vi "Load Plugin Action.vi"(7 "plugin path":path, 8 "error in (no error)":errorcluster, 9 "Unique Name":string, 10 "Plugin":T1, 11 "Launcher in":refnum<class "CIFPluginManager.lvclass">) -> (0 "error out":errorcluster, 3 "Launcher out":refnum<class "CIFPluginManager.lvclass">)   [LabVIEW 2021, in "CIFPluginManager.lvclass"]
doc: "This performs the loading action using VI Server. Because this process can be slow it is moved outside of the Load Plugin Prepare process. The prepare will detect most common configuration errors. This allows the UI to get any configuration errors returned but not need to wait for the full load to complete."
uses:
  CIFPluginManager.lvclass
  typedef/Discovered Plugin.ctl
  CIFCore/Common/Typedef/Version.ctl
  typedef/Plugin Metadata.ctl
  typedef/Plugin Management Data.ctl
  <vilib>/gRPC/LabVIEW gRPC Library/Shared/grpcId.ctl
  gRPC/CIF_Manager_server/RPC Messages/cif_plugincore_StatusData.ctl
  gRPC/CIF_Manager_server/RPC Messages/cif_plugincore_StatusData_State.ctl
  gRPC/CIF_Manager_server/RPC Messages/cif_plugincore_TimingStatistics.ctl
  gRPC/CIF_Manager_server/RPC Messages/cif_common_TimingStats.ctl
  gRPC/CIF_Manager_server/RPC Messages/cif_plugincore_FifoStatistics.ctl
  gRPC/CIF_Manager_server/RPC Messages/cif_plugincore_Error.ctl
  gRPC/CIF_Manager_server/RPC Messages/cif_plugincore_MonitorDoubles.ctl
  gRPC/CIF_Manager_server/RPC Messages/cif_plugincore_MonitorU64.ctl
  gRPC/CIF_Manager_server/RPC Messages/cif_plugincore_MonitorI64.ctl
  CIFPluginManager.lvclass/CIFPluginManager.ctl
  <vilib>/CIF Foundation/CIF Utilities/Time/System Time/LabVIEW Time to TAI Time.vi
  CIFCore/Common/CIFCoreCommon.lvlib
  <vilib>/gRPC/LabVIEW gRPC Library/grpc-lvsupport-release.lvlib
  gRPC/CIF_Manager_server/CIF_Manager_server.lvlib
  <vilib>/CIF Foundation/CIF Utilities/Time/Time_CIF_U.lvlib
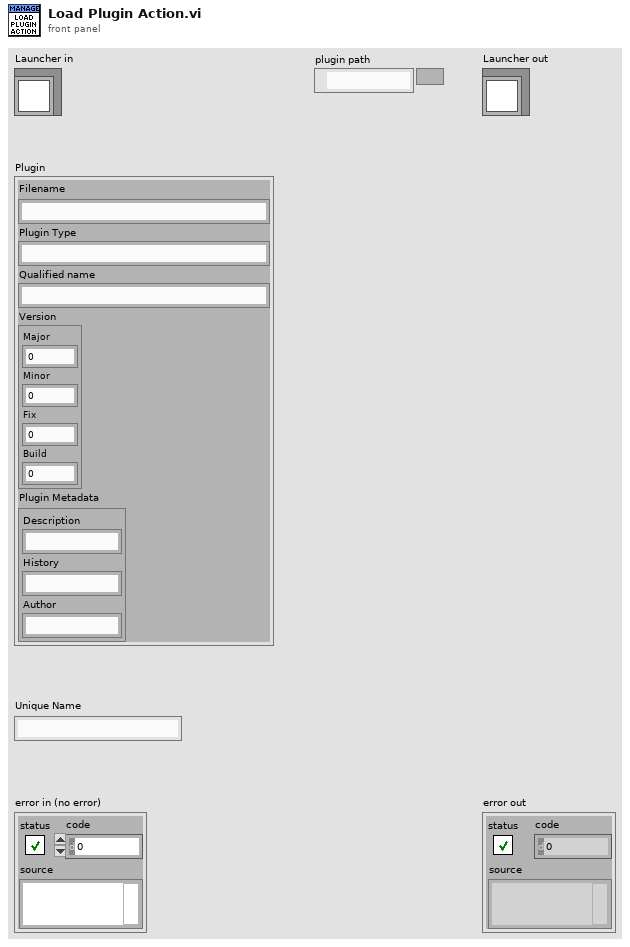
[diagram p1: front panel]
types:
  T1 = typedef "CIFPluginManager.lvclass/Discovered Plugin.ctl" = cluster{"Filename":string, "Plugin Type":string, "Qualified name":string, "Version":T2, "Plugin Metadata":T3}
  T2 = typedef "CIFCoreCommon.lvlib/Version.ctl" = cluster{"Major":i32, "Minor":i32, "Fix":i32, "Build":i32}
  T3 = typedef "CIFPluginManager.lvclass/Plugin Metadata.ctl" = cluster{"Description":string, "History":string, "Author":string}
  T4 = typedef "CIFPluginManager.lvclass/Plugin Management Data.ctl" = cluster{"vi reference":refnum<vi>, "gRPC ID":T5, "Plugin Type":string, "Unique Name":string, "gRPC Port":i32, "Version":T2, "Load Timestamp":i64, "Unload Timestamp":i64, "Unloading":bool, "Ready for removal":bool, "status":T6}
  T5 = typedef "grpc-lvsupport-release.lvlib/grpcId.ctl" = u64
  T6 = typedef "CIF_Manager_server.lvlib/cif_plugincore_StatusData.ctl" = cluster{"state":T7, "timing_statistics":T8, "fifo_statistics":T10, "error":T11, "monitor_doubles":T12, "monitor_u64s":T13, "monitor_i64s":T14}
  T7 = typedef "CIF_Manager_server.lvlib/cif_plugincore_StatusData_State.ctl" = enum32{"NULL", "CREATING", "LISTENING", "RUNNING", "CLEANINGUP", "DESTROYING"}
  T8 = typedef "CIF_Manager_server.lvlib/cif_plugincore_TimingStatistics.ctl" = cluster{"period":T9, "wake_error":T9, "execute":T9, "housekeep":T9, "idle":T9, "cleanup":T9, "custom_1":T9, "custom_2":T9}
  T9 = typedef "CIF_Manager_server.lvlib/cif_common_TimingStats.ctl" = cluster{"max":i64, "min":i64, "avg":dbl}
  T10 = typedef "CIF_Manager_server.lvlib/cif_plugincore_FifoStatistics.ctl" = cluster{"from_t0":T9, "from_previous_plugin":T9, "output_error":T9}
  T11 = typedef "CIF_Manager_server.lvlib/cif_plugincore_Error.ctl" = cluster{"status":bool, "code":i32}
  T12 = typedef "CIF_Manager_server.lvlib/cif_plugincore_MonitorDoubles.ctl" = cluster{"double_1":dbl, "double_2":dbl, "double_3":dbl, "double_4":dbl}
  T13 = typedef "CIF_Manager_server.lvlib/cif_plugincore_MonitorU64.ctl" = cluster{"u64_1":u64, "u64_2":u64, "u64_3":u64, "u64_4":u64}
  T14 = typedef "CIF_Manager_server.lvlib/cif_plugincore_MonitorI64.ctl" = cluster{"i64_1":i64, "i64_2":i64, "i64_3":i64, "i64_4":i64}
  T15 = typedef "Plugin Management Data Map.ctl" = map{string, T4}
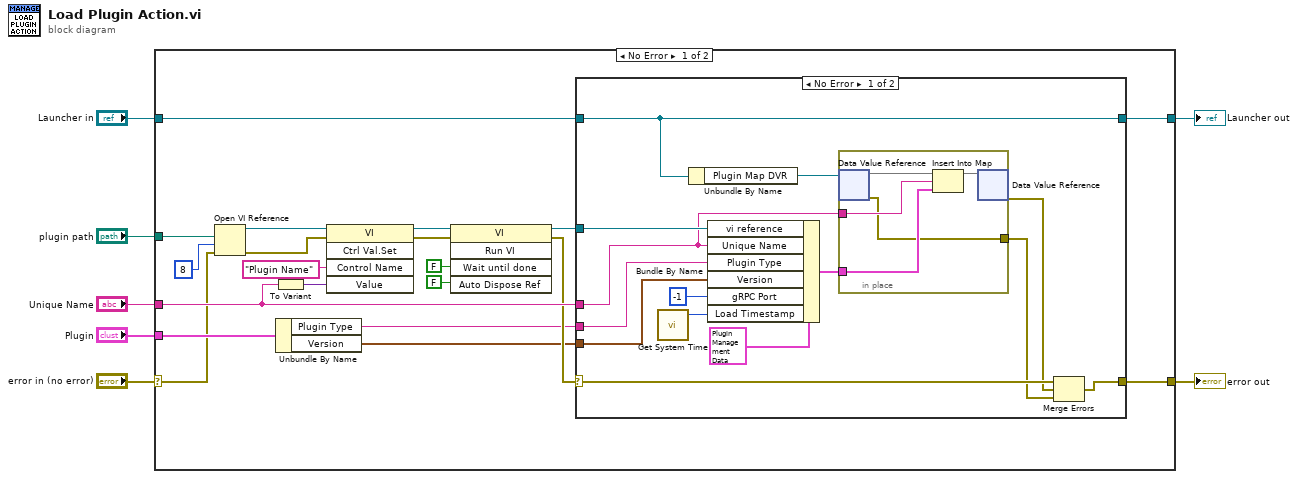
[diagram p0: block diagram]
diagram:
  n1 = case shown="No Error" "error in (no error)" {
    selector: "error in (no error)" -> [w22 w50]
    tunnel: [w27 w50] -> w6
    tunnel: [w26 w49] -> w4
    tunnel: "Launcher in" -> [w21 w49]
    tunnel: "Unique Name" -> [w25 _]
    tunnel: "plugin path" -> [w24 _]
    tunnel: "Plugin" -> [w23 _]
    frame No Error {
      n2 = Open VI Reference(vi path=w24, options=8, error in (no error)=w22) -> (vi reference=w15:refnum<vi>, error out=w18:errorcluster)  [unwired: 3 in]
      n3 = To Variant(anything=w25) -> (Variant=w13:variant)
      n4 = Unbundle By Name(w23) -> ("Plugin Type"=w9:string, "Version"=w8:T2)
      n5 = invoke class="VI" method="Ctrl Val.Set"(reference=w15, error in=w18, "Control Name"="Plugin Name", "Value"=w13) -> (reference out=w17:refnum<vi>, error out=w16:errorcluster)  [unwired: 1 in, 3 out]
      n6 = invoke class="VI" method="Run VI"(reference=w17, error in=w16, "Wait until done"=FALSE ("Wait Until Done"), "Auto Dispose Ref"=FALSE ("Auto Dispose Reference")) -> (reference out=w10:refnum<vi>, error out=w11:errorcluster)  [unwired: 1 in, 3 out]
      n7 = case shown="No Error" w11 {
        selector: w11 -> [w31 w47]
        tunnel: w10 -> [w41 _]
        tunnel: w25 -> [w38 _]
        tunnel: w21 -> [w33 w48]
        tunnel: [w28 w47] -> w27
        tunnel: w9 -> [w39 _]
        tunnel: [w33 w48] -> w26
        tunnel: w8 -> [w36 _]
        frame No Error {
          n8 = call <vilib>:"Get System Time.vi"() -> ("Time (ns)"=w34:i64)  [unwired: 5 in]
          n9 = Unbundle By Name(w33) -> ("Plugin Map DVR"=w32:refnum<data-value>)
          n10 = Bundle By Name(cluster=T4 {"vi reference"=refnum, "gRPC ID"=0, "Plugin Type"="", "Unique Name"="", "gRPC Port"=0, "Version"={"Major"=0, "Minor"=0, "Fix"=0, "Build"=0}, "Load Timestamp"=0, "Unload Timestamp"=0, "Unloading"=FALSE, "Ready for removal"=FALSE, "status"={"state"=enum."NULL", "timing_statistics"={"period"={"max"=0, "min"=0, "avg"=0.0}, "wake_error"={"max"=0, "min"=0, "avg"=0.0}, "execute"={"max"=0, "min"=0, "avg"=0.0}, "housekeep"={"max"=0, "min"=0, "avg"=0.0}, "idle"={"max"=0, "min"=0, "avg"=0.0}, "cleanup"={"max"=0, "min"=0, "avg"=0.0}, "custom_1"={"max"=0, "min"=0, "avg"=0.0}, "custom_2"={"max"=0, "min"=0, "avg"=0.0}}, "fifo_statistics"={"from_t0"={"max"=0, "min"=0, "avg"=0.0}, "from_previous_plugin"={"max"=0, "min"=0, "avg"=0.0}, "output_error"={"max"=0, "min"=0, "avg"=0.0}}, "error"={"status"=FALSE, "code"=0}, "monitor_doubles"={"double_1"=0.0, "double_2"=0.0, "double_3"=0.0, "double_4"=0.0}, "monitor_u64s"={"u64_1"=0, "u64_2"=0, "u64_3"=0, "u64_4"=0}, "monitor_i64s"={"i64_1"=0, "i64_2"=0, "i64_3"=0, "i64_4"=0}}} ("Plugin Management Data"), "vi reference"=w41, "Unique Name"=w38, "Plugin Type"=w39, "Version"=w36, "gRPC Port"=-1, "Load Timestamp"=w34) -> (w37:T4)
          n11 = in-place {
            in-place-border: w38 -> [w46]
            in-place-border: w37 -> [w45]
            in-place-border: [w42] -> w30
            n12 = in-place-dvr #1(w32) -> (w44:T15, w42:errorcluster)
            n13 = Insert Into Map(map in=w44, key=w46, value=w45) -> (map out=w43:T15)  [unwired: 2 out]
            n14 = in-place-dvr #1(w43) -> (w29:errorcluster)  [unwired: 1 out]
          }
          n15 = Merge Errors(w31, w29, w30) -> (w28:errorcluster)
        }
        frame Error {
        }
      }
    }
    frame Error {
    }
  }
  "error out" <- w6
  "Launcher out" <- w4
